vi "CheckLockAndSaveClass.vi"(8 "error in (no error)":errorcluster, 11 "LVClass ref":refnum<vi>) -> (0 "error out":errorcluster, 3 "LVClass ref":refnum<vi>)   [LabVIEW 2019, in "BlueUtilityScripts.lvlib"]
uses:
  BlueUtilityScripts.lvlib
  <vilib>/Utility/error.llb/Error Cluster From Error Code.vi
  <vilib>/ErrorRing/Error Ring.xnode
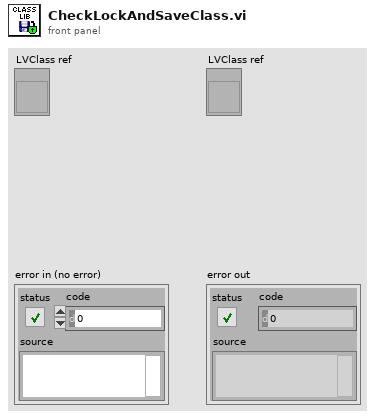
[diagram p1: front panel]
types:
  T1 = enum32{"invalid lock state", "Not Locked", "Locked (No Password)", "Password-protected"}
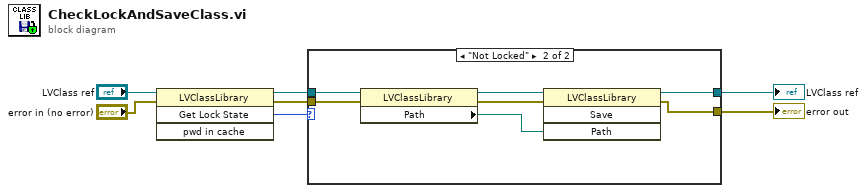
[diagram p0: block diagram]
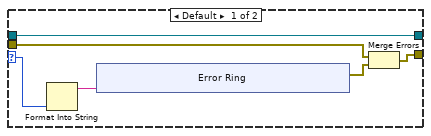
[diagram p2: hidden frame]
diagram:
  n1 = invoke class="LVClassLibrary" method="Get Lock State"(reference="LVClass ref", error in="error in (no error)") -> (reference out=w3:refnum<vi>, error out=w2:errorcluster, "Get Lock State"=w1:T1)  [unwired: 2 in, 1 out]
  n2 = case shown="\"Not Locked\"" w1 {
    selector: w1 -> [w12 _]
    tunnel: [w13 w24] -> w7
    tunnel: [w8 w23] -> w6
    tunnel: w3 -> [w13 w22]
    tunnel: w2 -> [w10 w21]
    frame Default {
      n3 = Format Into String(w12) -> (resulting string=w11:string)  [unwired: 3 in, 1 out]
      n4 = xnode "Error Ring"("parameter 0"=w11) -> ("error out"=w9:errorcluster)
      n5 = Merge Errors(w10, w9) -> (w8:errorcluster)
    }
    frame "Not Locked" {
      n6 = property class="LVClassLibrary"(reference=w22, error in=w21) -> (reference out=w27:refnum<vi>, error out=w25:errorcluster, "Path"=w26:path)
      n7 = invoke class="LVClassLibrary" method="Save"(reference=w27, error in=w25, "Path"=w26) -> (reference out=w24:refnum<vi>, error out=w23:errorcluster)  [unwired: 1 in, 2 out]
    }
  }
  "error out" <- w6
  "LVClass ref" <- w7
